vi "Firmware.vi"() -> ()   [LabVIEW 2026]
panel:
  in  "Ayuda":bool
  in  "Stop Button":bool
  in  "Install":bool
  # "LV_ESP32 - Instalador de Firmware"
  # "Arduino + Labview = instrumentacion virtual Low cost"
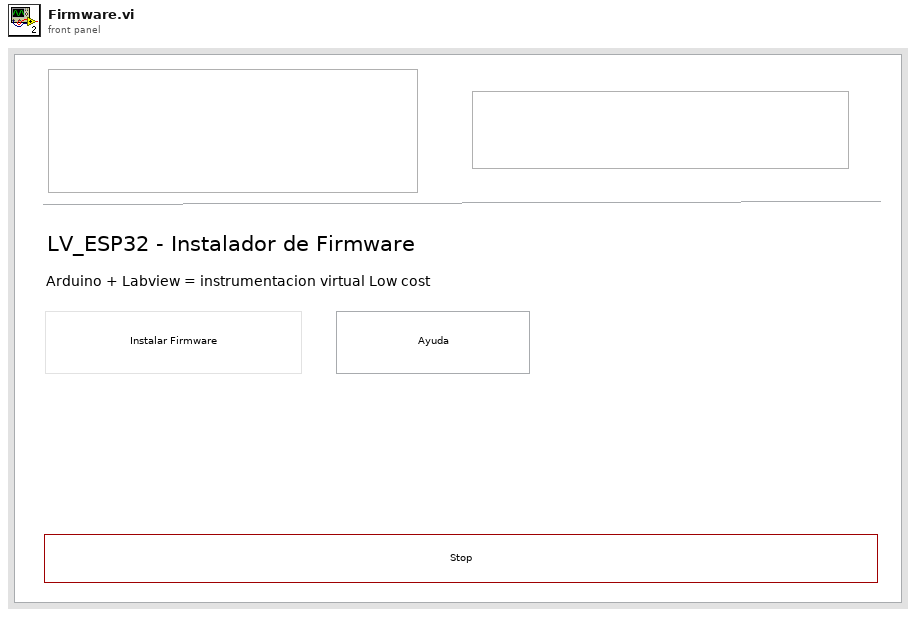
[diagram p1: front panel]
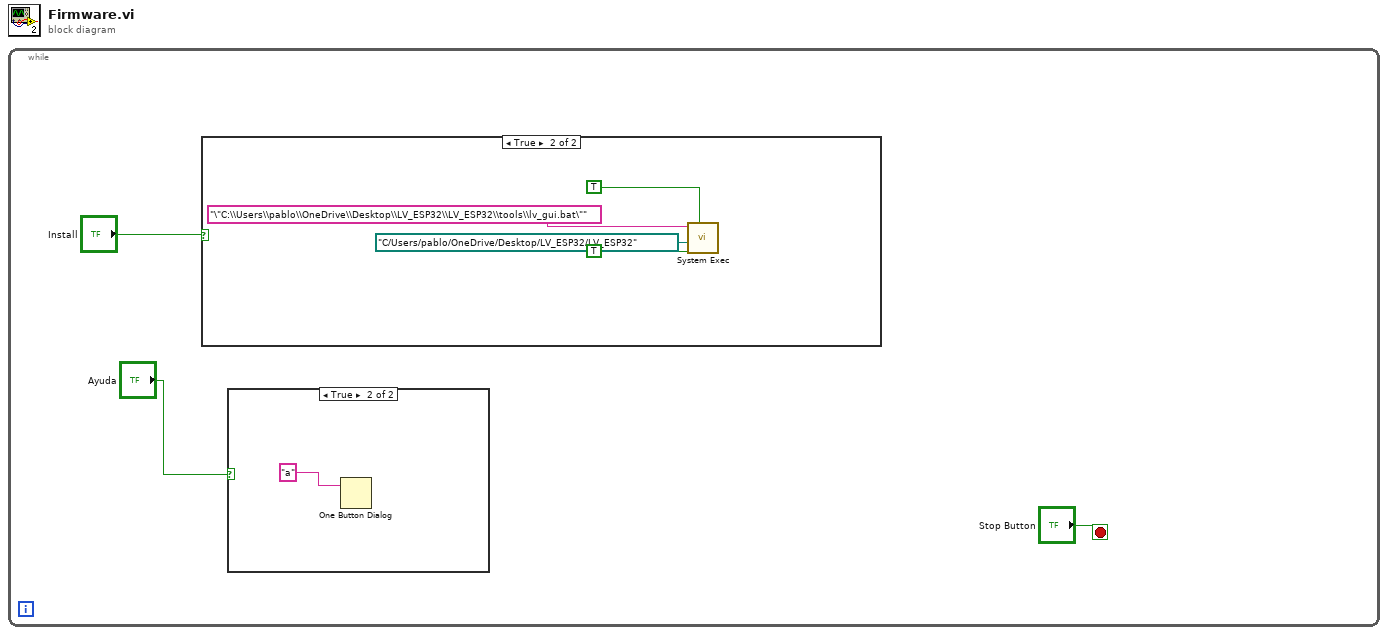
[diagram p0: block diagram]
diagram:
  n1 = while {
    stop <- "Stop Button" stop-if-true
    n2 = case shown="True" "Install" {
      frame False {
      }
      frame True {
        n3 = call <vilib>:"System Exec.vi"("run minimized? (F)"=TRUE, "wait until completion? (T)"=TRUE, "working directory"=path "C:/Users/pablo/OneDrive/Desktop/LV_ESP32/LV_ESP32", "command line"="\"C:\\Users\\pablo\\OneDrive\\Desktop\\LV_ESP32\\LV_ESP32\\tools\\lv_gui.bat\"") -> ()  [unwired: 4 in, 4 out]
      }
    }
    n4 = case shown="True" "Ayuda" {
      frame False {
      }
      frame True {
        n5 = One Button Dialog(message="a") -> ()  [unwired: 1 in, 1 out]
      }
    }
  }
